vi "Do Core.vi"(8 "error in":errorcluster, 9 "Actor in":refnum<class "Actor.lvclass">, 11 "Perform Action Msg in":refnum<class "Perform Action Msg.lvclass">) -> (0 "error out":errorcluster, 1 "Actor out":refnum<class "Actor.lvclass">, 2 "Output":variant)   [LabVIEW 2023, in "IMSS Target Actor.lvlib" / "Perform Action Msg.lvclass"]
uses:
  Perform Action Msg.lvclass
  <vilib>/ActorFramework/Actor/Actor.lvclass
  IMSS Target Actor/IMSS Target Actor.lvclass
  Perform Action Msg.lvclass/Perform Action Msg.ctl
  1cf320dd-9f96-48fa-8e4c-b9a4ae22bce5.vi
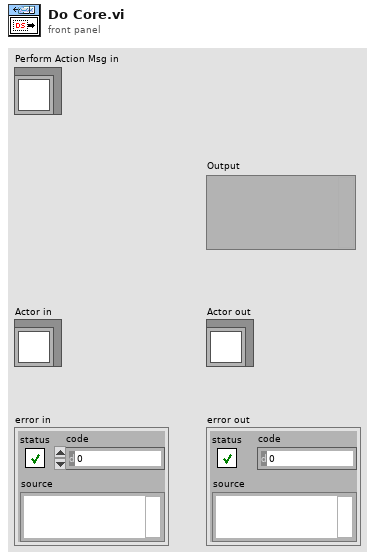
[diagram p1: front panel]
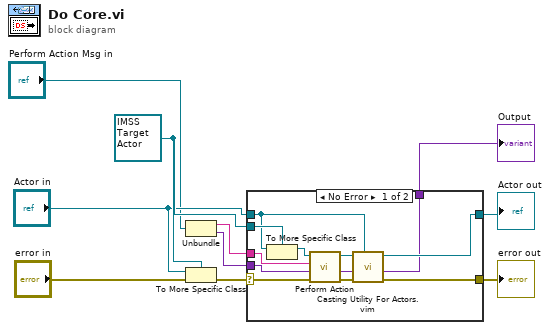
[diagram p0: block diagram]
diagram:
  w9 = refnum<class "IMSS Target Actor.lvclass"> refnum ("Actor in")
  n1 = Unbundle("Perform Action Msg in") -> (w8:string, w7:variant)
  n2 = To More Specific Class(target class=w9, reference="Actor in", error in="error in") -> (error out=w10:errorcluster)  [unwired: 1 out]
  n3 = case shown="No Error" w10 {
    selector: w10 -> [w21 w23]
    tunnel: [w15 w23] -> w5
    tunnel: [w16 w22] -> w4
    tunnel: "Actor in" -> [w18 w22]
    tunnel: w9 -> [w19 _]
    tunnel: w8 -> [w13 _]
    tunnel: w7 -> [w12 _]
    tunnel: [w11 _] -> w3
    frame No Error {
      n4 = To More Specific Class(target class=w19, reference=w18) -> (specific class reference=w20:refnum<class "IMSS Target Actor.lvclass">)  [unwired: 1 in, 1 out]
      n5 = call-dynamic "Perform Action.vi"("error in"=w21, "Input"=w12, "Task-Point Ident"=w13, "IMSS Target Actor in"=w20) -> ("error out"=w14:errorcluster, "Output"=w11:variant, "IMSS Target Actor out"=w17:refnum<class "IMSS Target Actor.lvclass">)  [unwired: 5 in]
      n6 = call "Casting Utility For Actors.vim"("type"=w18, "error in (no error)"=w14, "Actor in"=w17) -> ("error out"=w15:errorcluster, "Actor out"=w16:refnum<class "Actor.lvclass">)  [unwired: 7 in]
    }
    frame Error {
      # "If type check fails, pass the original object out again."
    }
  }
  "error out" <- w5
  "Actor out" <- w4
  "Output" <- w3
